vi "RunPhoenix.vi"() -> ()   [LabVIEW 2020]
uses:
  Controls/ComUDP.ctl
  Controls/vision_control.ctl
panel:
  out "com":T1={"UDP GrSim TX"=TRUE, "Address:"="127.0.0.1", "Port:"=20011}
  out "referee":T2
  out "vision":T2
  in  "SSL UDP RX":T2={"Local IP:"="", "Port"=10020, "Server IP:"="224.5.23.2"}
  in  "RefBox UDP RX":T2={"Local IP:"="10.100.62.227", "Port"=10003, "Server IP:"="224.5.23.1"}
  in  "Com UDP":T1={"UDP GrSim TX"=TRUE, "Address:"="127.0.0.1", "Port:"=20011}
  out "SSL RX":bool
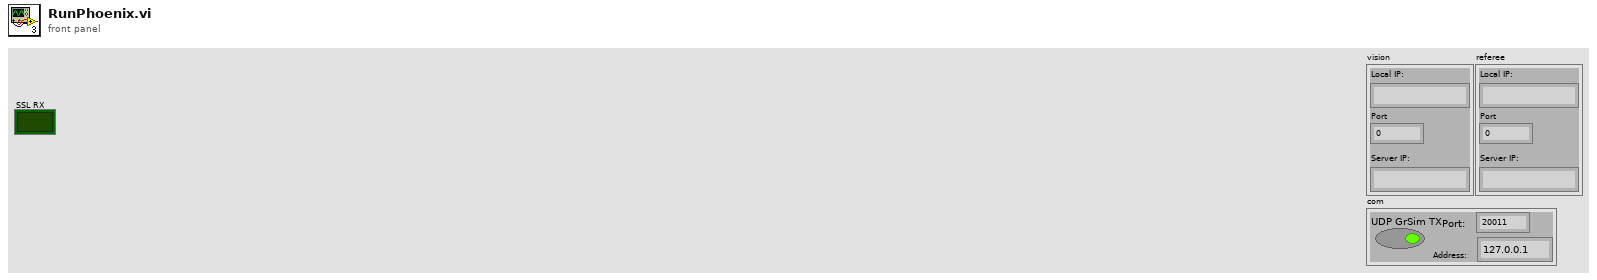
[diagram p1: front panel]
types:
  T1 = typedef "ComUDP.ctl" = cluster{"UDP GrSim TX":bool, "Address:":string, "Port:":u16}
  T2 = typedef "vision_control.ctl" = cluster{"Local IP:":string, "Port":i32, "Server IP:":string}
  T3 = enum32{"Invalid", "Standard", "Closed", "Hidden", "Minimized", "Maximized"}
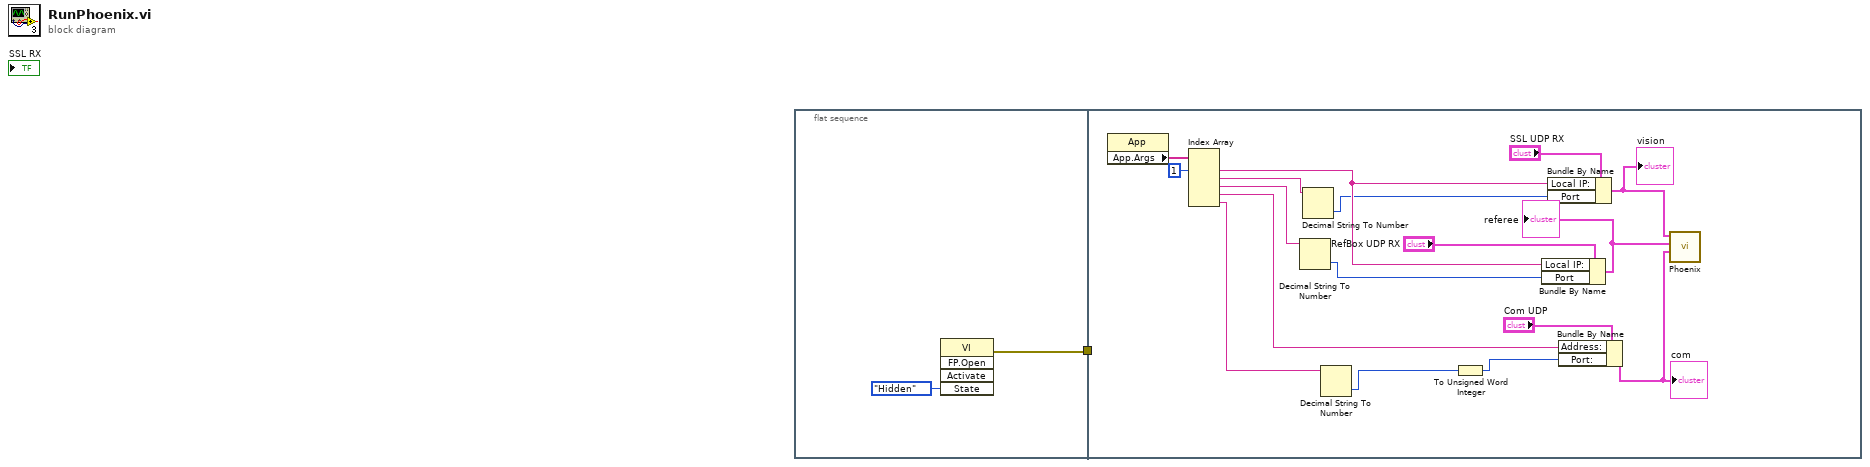
[diagram p0: block diagram]
diagram:
  n1 = flat-sequence {
    tunnel: [w2] -> w1
    tunnel: w1 -> [_]
    frame #0 {
      n2 = invoke class="VI" method="FP.Open"("State"=T3."Hidden") -> (error out=w2:errorcluster)  [unwired: 4 in, 4 out]
    }
    frame #1 {
      n3 = property class="App"() -> ("App.Args"=w17:string[])  [unwired: 2 in, 2 out]
      n4 = Index Array(array=w17, index #1=1 ("index")) -> (element #1=w15:string, element #2=w14:string, element #3=w12:string, element #4=w10:string, element #5=w9:string)  [unwired: 4 in]
      n5 = Decimal String To Number(string=w12) -> (number=w11:i32)  [unwired: 2 in, 1 out]
      n6 = Decimal String To Number(string=w14) -> (number=w13:i32)  [unwired: 2 in, 1 out]
      n7 = Decimal String To Number(string=w9) -> (number=w7:i32)  [unwired: 2 in, 1 out]
      n8 = To Unsigned Word Integer(number=w7) -> (unsigned 16bit integer=w8:u16)
      n9 = Bundle By Name(cluster="RefBox UDP RX", "Local IP:"=w15, "Port"=w11) -> (w5:T2)
      "referee" <- w5
      n10 = Bundle By Name(cluster="SSL UDP RX", "Local IP:"=w15, "Port"=w13) -> (w6:T2)
      "vision" <- w6
      n11 = Bundle By Name(cluster="Com UDP", "Address:"=w10, "Port:"=w8) -> (w4:T1)
      "com" <- w4
      n12 = call "Phoenix.vi"("Com UDP"=w4, "RefBox UDP RX"=w5, "SSL UDP RX"=w6) -> ()  [unwired: 9 in]
    }
  }
